vi "PowerCalibration.vi"() -> ()   [LabVIEW 2017]
uses:
  <vilib>/express/express analysis/Spectral/Block/exnSpectralBlock spectral measurements RMS poly.vi
  <vilib>/express/express analysis/Spectral/Block/exnSpectralBlock spectral measurements RMS DDT.vi
  <vilib>/express/express analysis/Spectral/XNode/ExpressSpectralMeasurementsBlockNode.xnode
panel:
  out "Waveform Graph 2":dynamicdata(graph)
  out "Waveform Graph":dynamicdata(graph)
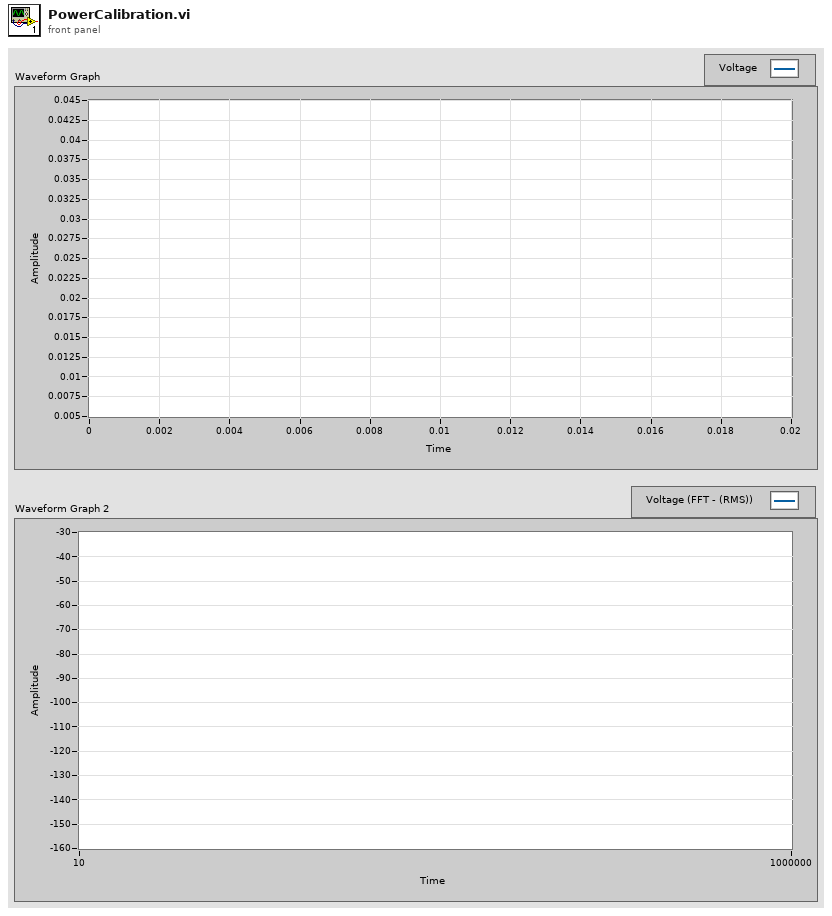
[diagram p1: front panel]
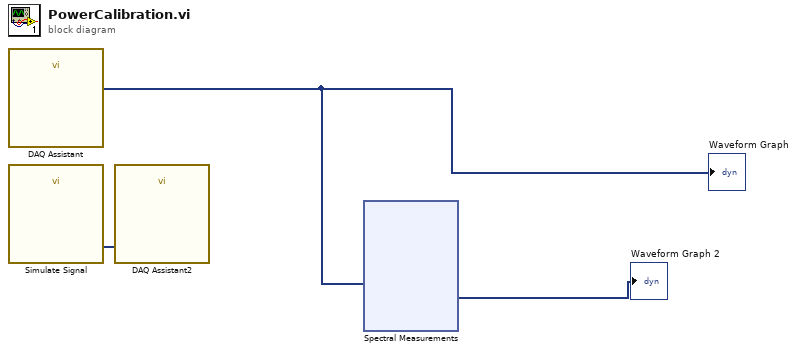
[diagram p0: block diagram]
diagram:
  n1 = call "DAQ Assistant"() -> ("data"=w2:dynamicdata)  [unwired: 17 in, 2 out]
  "Waveform Graph" <- w2
  n2 = call "Simulate Signal"() -> ("Sine"=w3:dynamicdata)  [unwired: 14 in, 1 out]
  n3 = call "DAQ Assistant2"("data"=w3) -> ()  [unwired: 17 in, 2 out]
  n4 = xnode "Spectral Measurements"("Signals"=w2) -> ("FFT - (RMS)"=→"Waveform Graph 2":dynamicdata)  [unwired: 1 in, 2 out]
